vi "AB_Log_NewBuild.vi"(8 "error in (no error)":errorcluster, 11 "Object":T1) -> (0 "error out":errorcluster)   [LabVIEW 2020]
uses:
  <resource>/Framework/Providers/API/ItemRef.ctl
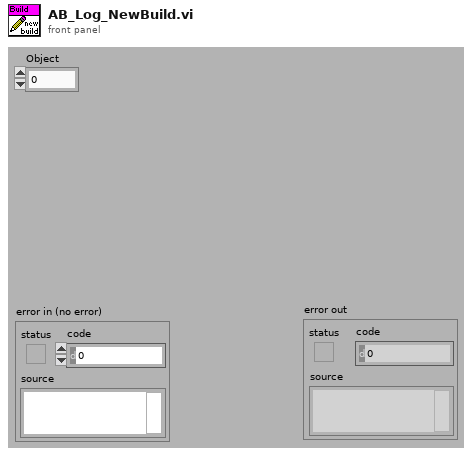
[diagram p1: front panel]
types:
  T1 = typedef "ItemRef.ctl" = u64
  T2 = typedef "AB_RW_Project_Build_Data.ctl" = cluster{"buildSpecName":string, "buildSpecDescription":string, "excludeTypedefs":bool, "excludePolymorphicVIs":bool, "excludeLibraryItems":bool, "modifyLibraryFile":bool, "defaultLanguage":string, "supportedLanguages":string[], "excludedDirectories":path[], "userLog_Path":path, "preActionVIID":string, "postActionVIID":string, "localDest_Path":path, "targetDest_Path":path, "removeVIObject":u16, "previewCache_ID":string, "buildCache_ID":string, "excludeInlineSubVIs":bool, "bldVersion":cluster{"major":u16, "minor":u16, "patch":u16, "build":u16}, "autoIncrement":bool, "excludeDependentPPLs":bool, "excludeDependentDLLs":bool}
  T3 = enum32{"invalid OS target", "Mac OS", "Windows 3.1", "Windows 95/NT", "Solaris 1", "Solaris 2", "HP-UX", "PowerMAX", "Linux", "Irix", "Rhapsody", "BeOS", "AIX", "OSF1", "VxWorks", "PharLap", "Carbon", "RTX", "Windows x64", "Linux x64", "Mac OS X x64"}
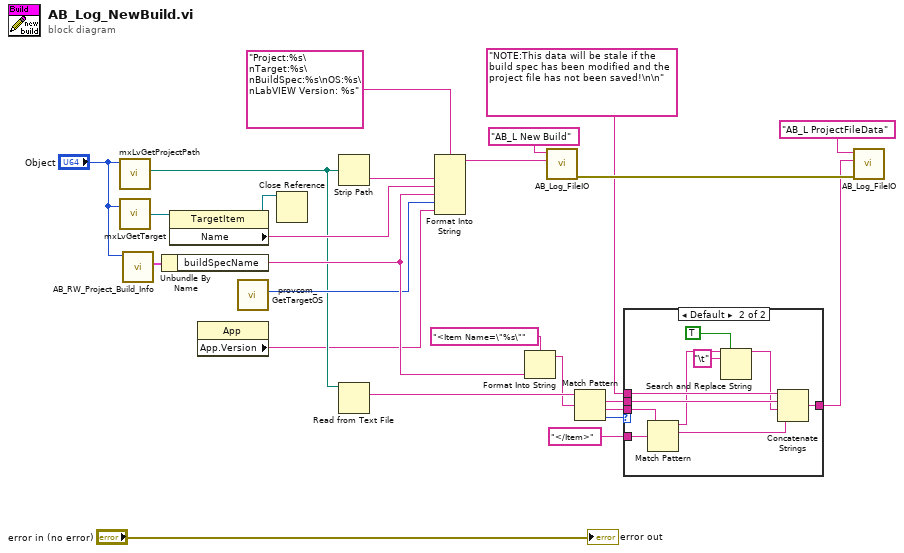
[diagram p0: block diagram]
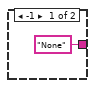
[diagram p2: hidden frame]
diagram:
  n1 = call <resource>:"mxLvGetProjectPath.vi"("Item"="Object") -> ("Project Path"=w2:path)  [unwired: 8 in, 2 out]
  n2 = call <resource>:"mxLvGetTarget.vi"("Item"="Object") -> ("Target"=w24:refnum<vi>)  [unwired: 1 in, 2 out]
  n3 = call <vilib>:"AB_RW_Project_Build_Info.vi"("Object In"="Object") -> ("buildInfo out"=w20:T2)  [unwired: 8 in, 2 out]
  n4 = Unbundle By Name(w20) -> ("buildSpecName"=w15:string)
  n5 = property class="TargetItem"(reference=w24) -> (reference out=w11:refnum<vi>, "Name"=w21:string)  [unwired: 1 in, 1 out]
  n6 = property class="App"() -> ("App.Version"=w1:string)  [unwired: 2 in, 2 out]
  n7 = call <resource>:"provcom_GetTargetOS.vi"() -> ("App.TargetOS"=w4:T3)  [unwired: 11 in]
  n8 = Close Reference(reference=w11) -> ()  [unwired: 1 in, 1 out]
  n9 = Strip Path(path=w2) -> (name=w22:string)  [unwired: 1 out]
  n10 = Read from Text File(file (use dialog)=w2) -> (text=w14:string)  [unwired: 3 in, 3 out]
  n11 = Format Into String(format string="Project:%s\nTarget:%s\nBuildSpec:%s\nOS:%s\nLabVIEW Version: %s", w22, w21, w15, w4, w1) -> (resulting string=w10:string)  [unwired: 2 in, 1 out]
  n12 = Format Into String(format string="<Item Name=\"%s\"" ("regular expression"), w15) -> (resulting string=w5:string)  [unwired: 2 in, 1 out]
  n13 = call <vilib>:"AB_Log_FileIO.vi"("data"=w10, "newSection"="AB_L New Build" ("data")) -> ("error out"=w13:errorcluster)  [unwired: 9 in]
  n14 = Match Pattern(string=w14, regular expression=w5) -> (match substring=w19:string, after substring=w17:string, offset past match=w6:i32)  [unwired: 1 in, 1 out]
  n15 = case shown="Default" w6 {
    tunnel: w19 -> [_ w35]
    tunnel: "</Item>" ("regular expression") -> [_ w34]
    tunnel: w17 -> [_ w33]
    tunnel: "NOTE:This data will be stale if the build spec has been modified and the project file has not been saved!\n\n" ("string") -> [_ w32]
    tunnel: ["None" w31] -> w8
    frame -1 {
    }
    frame Default {
      n16 = Match Pattern(string=w33, regular expression=w34) -> (before substring=w30:string, match substring=w36:string)  [unwired: 1 in, 2 out]
      n17 = Search and Replace String(replace all?=TRUE ("replace all? (F)"), input string=w30, search string="\t") -> (result string=w29:string)  [unwired: 5 in, 3 out]
      n18 = Concatenate Strings(w32, w35, w29, w36) -> (w31:string)
    }
  }
  n19 = call <vilib>:"AB_Log_FileIO.vi"("error in (no error)"=w13, "data"=w8, "newSection"="AB_L ProjectFileData" ("data")) -> ()  [unwired: 8 in, 1 out]
  "error out" <- "error in (no error)"
